vi "Self Alias.vi"(11 "Ex Event Actor in":refnum<class "Ex Event Actor.lvclass">) -> (2 "Self Alias":string)   [LabVIEW 2021, in "Ex Event Actor.lvlib" / "Ex Event Actor.lvclass"]
uses:
  Ex Event Actor.lvclass
  Ex Event Actor.lvclass/Ex Event Actor.ctl
  Actor/Event Actor/Event Actor.lvclass
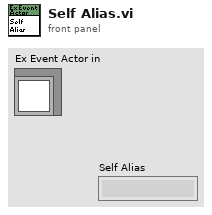
[diagram p1: front panel]
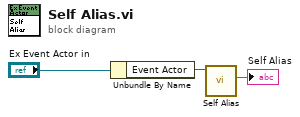
[diagram p0: block diagram]
diagram:
  n1 = Unbundle By Name("Ex Event Actor in") -> ("Event Actor"=w2:refnum<class "Event Actor.lvclass">)
  n2 = call-dynamic "Self Alias.vi"("Actor in"=w2) -> ("Self Alias"=→"Self Alias":string)  [unwired: 10 in]
